vi "CAENHV Get Ch Param Info.vi"(8 "error in (no error)":errorcluster, 9 "Ch":u16, 10 "slot":u16, 11 "handle":i32) -> (0 "error out":errorcluster, 2 "ParNumber":i32, 3 "ParNameList":string[](array[string]))   [LabVIEW 2018, in "CAENHVWrapper.lvlib"]
doc: "CAENHVLIB_API CAENHVRESULT CAENHV_GetChParamInfo(int handle, ushort slot, ushort Ch, char **ParNameList, int *ParNumber);"
uses:
  <instrlib>/CAENHVWrapper/CAENHVWrapper.lvlib
  <vilib>/Utility/importsl/GetValueByPointer/datatype.ctl
  <vilib>/Utility/importsl/GetValueByPointer/GetValueByPointer.xnode
  <instrlib>/CAENHVWrapper/VIs/CAENHVWrapper.dll
  <resource>/lvimptsl.dll
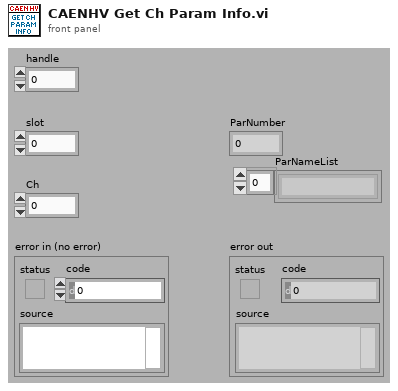
[diagram p1: front panel]
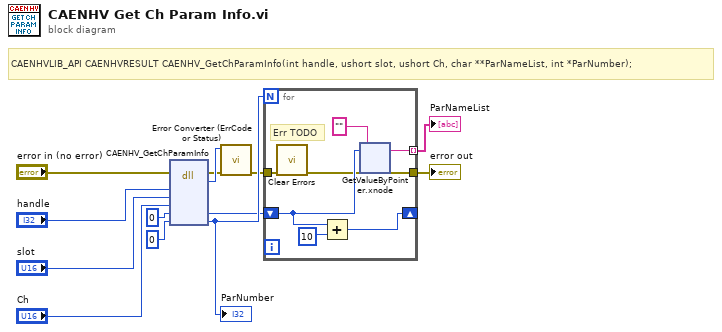
[diagram p0: block diagram]
diagram:
  # "CAENHVLIB_API CAENHVRESULT CAENHV_GetChParamInfo(int handle, ushort slot, ushort Ch, char **ParNameList, int *ParNumber);"
  n1 = dll-call lib="C:/Program Files (x86)/National Instruments/LabVIEW 2018/instr.lib/CAENHVWrapper/VIs/CAENHVWrapper.*" fn="CAENHV_GetChParamInfo"(error in="error in (no error)", "handle"="handle", "slot"="slot", "Ch"="Ch", "ParNameList"=i64 0, "ParNumber"=0) -> (error out=w7:errorcluster, "return type"=w8:i32, "ParNameList"=w3:i64, "ParNumber"=w4:i32)  [unwired: 5 in, 1 out]
  "ParNumber" <- w4
  n2 = call <instrlib>:"Error Converter (ErrCode or Status).vi"("error in (no error)"=w7, "error code"=w8) -> ("error out"=w1:errorcluster)  [unwired: 9 in]
  n3 = for {
    N: w4 -> [_]
    shift-right: [w17] -> _
    shift-left: w3 -> [w20]
    tunnel: [w21] -> w5
    tunnel: [w18] -> w2 mode=indexing
    tunnel: w1 -> [w15]
    # "Err TODO"
    n4 = call <vilib>:"Clear Errors.vi"("error in (no error)"=w15) -> ("error out"=w14:errorcluster)  [unwired: 5 in, 1 out]
    n5 = Add(x=w20, y=i64 10) -> (x+y=w17:i64)
    n6 = xnode "GetValueByPointer.xnode"("Pointer"=w20, "InputType"="", "ErrorIn"=w14) -> ("Output"=w18:string, "ErrorOut"=w21:errorcluster)  [unwired: 1 in]
  }
  "error out" <- w5
  "ParNameList" <- w2
